vi "Find Workspace.vi"(8 "Error In":errorcluster, 9 "Assembly Type":string, 10 "Control In":T2={"I-O.lvclass"=refnum, "Gantry"=refnum, "Dispenser"="COM1"}, 11 "Workspace In":refnum<class "Fixture.lvclass">) -> (0 "Error Out":errorcluster, 1 "Workspace Out":T1, 2 "Control Out":T2={"I-O.lvclass"=refnum, "Gantry"=refnum, "Dispenser"="COM1"}, 3 "Workspace Out":refnum<class "Fixture.lvclass">)   [LabVIEW 2021, in "Fixture.lvclass"]
uses:
  Fixture.lvclass
  Controller/Controllers.ctl
  Controller/I-O/I-O.lvclass
  C:/Program Files (x86)/Aerotech/A3200/LabVIEW/2010/Bin/Aerotech.A3200.dll
  Program Files (x86)/Aerotech/A3200/LabVIEW/2010/Bin/Aerotech.A3200.dll
  Workspace.ctl
  Fixture.lvclass/Fixture.ctl
  Controller/Controller.lvclass
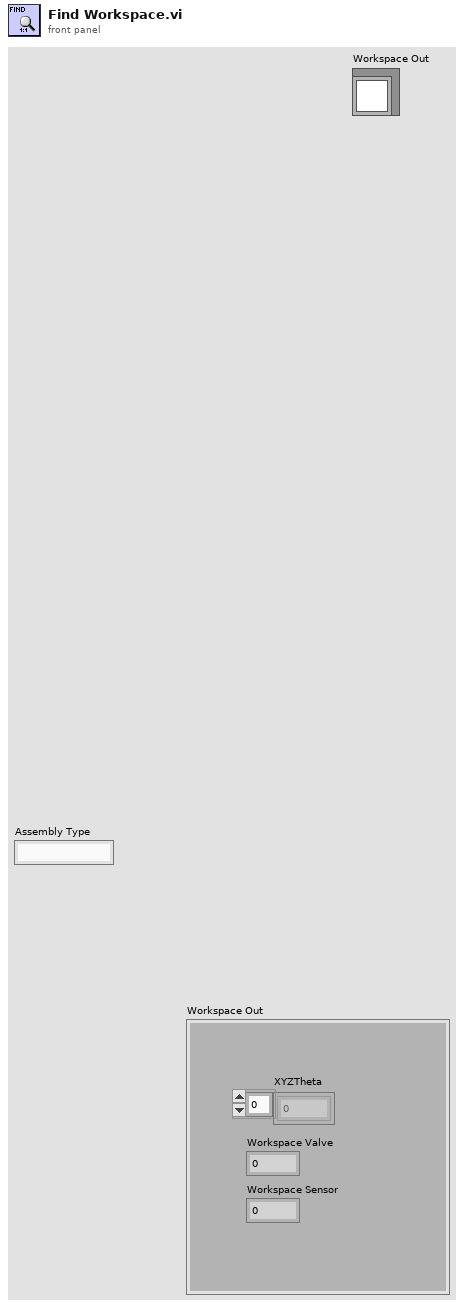
[diagram p1: front panel]
types:
  T1 = typedef "Fixture.lvclass/Workspace.ctl" = cluster{"XYZTheta":dbl[], "Workspace Valve":i32, "Workspace Sensor":i32}
  T2 = typedef "Controller.lvclass/Controllers.ctl" = cluster{"I-O.lvclass":refnum<class "I-O.lvclass">, "Gantry":refnum<k24>, "Dispenser":refnum<visa-resource-name>}
  T3 = typedef "I-O.lvclass/Pin Map.ctl" = cluster{"Region Valves":i32[], "Extra Valves":dbl[][][], "Tool Primary Valve":i32, "Tool Secondary Valve":i32, "Region Sensors":i32[], "Extra Sensors":dbl[][][], "Tool Primary Sensor":dbl, "Tool Secondary Sensor":dbl, "Compression Sensor":dbl, "5V":i32, "Dispenser Sensor":dbl}
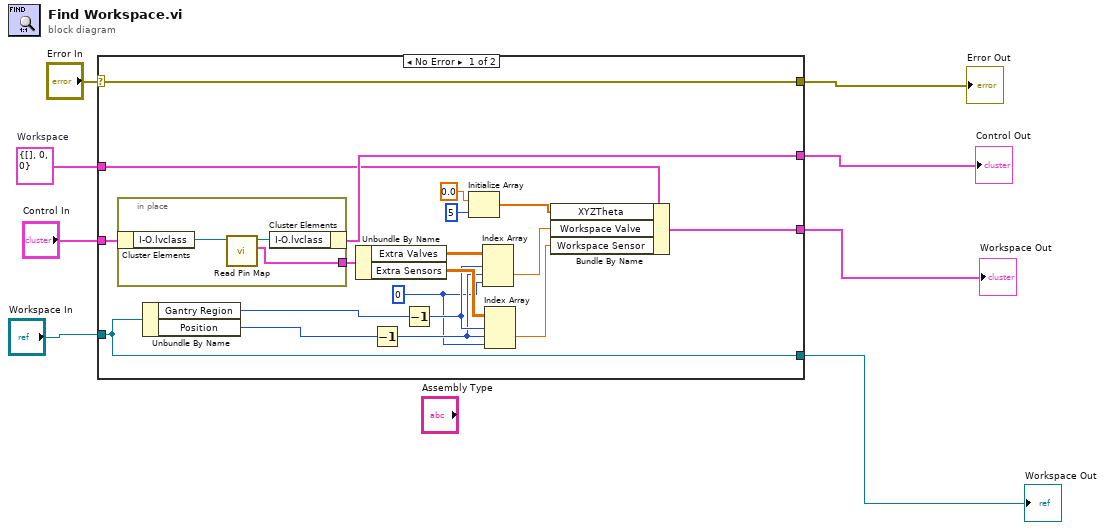
[diagram p0: block diagram]
diagram:
  w4 = T1 {"XYZTheta"=[], "Workspace Valve"=0, "Workspace Sensor"=0}  # Workspace
  n1 = case shown="No Error" "Error In" {
    selector: "Error In" -> [w27 w34]
    tunnel: [w27 w34] -> w7
    tunnel: [w22 w33] -> w5
    tunnel: "Workspace In" -> [w22 w33]
    tunnel: w4 -> [w14 w32]
    tunnel: [w16 w32] -> w3
    tunnel: "Control In" -> [w26 w31]
    tunnel: [w25 w31] -> w1
    frame No Error {
      w9 = 0
      n2 = in-place {
        in-place-border: [w28] -> w21
        n3 = in-place-cluster #1(w26) -> ("I-O.lvclass"=w30:refnum<class "I-O.lvclass">)
        n4 = call-dynamic "Read Pin Map.vi"("I-O in"=w30) -> ("Pin Map 2"=w28:T3, "I-O out"=w29:refnum<class "I-O.lvclass">)  [unwired: 8 in, 1 out]
        n5 = in-place-cluster #1("I-O.lvclass"=w29) -> (w25:T2)
      }
      n6 = Unbundle By Name(w22) -> ("Gantry Region"=w13:i32, "Position"=w11:i32)
      n7 = Unbundle By Name(w21) -> ("Extra Valves"=w20:dbl[][][], "Extra Sensors"=w19:dbl[][][])
      n8 = Decrement(x=w11) -> (x-1=w10:i32)
      n9 = Decrement(x=w13) -> (x-1=w12:i32)
      n10 = Initialize Array "Initialize Array"(0.0 ("element"), 5 ("dimension size")) -> (w15:dbl[])
      n11 = Index Array(array=w20, index (dim 0)=w12, index (dim 1)=w10, index (dim 2)=w9) -> (element=w18:dbl)
      n12 = Index Array "Index Array"(array=w19, index (dim 0)=w12, index (dim 1)=w10, index (dim 2)=w9) -> (element=w17:dbl)
      n13 = Bundle By Name(cluster=w14, "XYZTheta"=w15, "Workspace Valve"=w18, "Workspace Sensor"=w17) -> (w16:T1)
    }
    frame Error {
    }
  }
  "Error Out" <- w7
  "Workspace Out" <- w5
  "Control Out" <- w1
  "Workspace Out" <- w3
